vi "DSB Modulation PLL for Graph.vi"() -> ()   [LabVIEW 2013]
uses:
  <vilib>/sound2/lvsound2.llb/Sound File Info (path).vi
  <vilib>/sound2/lvsound2.llb/Sound File Read Open.vi
  <vilib>/sound2/lvsound2.llb/Sound File Read (DBL).vi
  <vilib>/Waveform/WDTOps.llb/WDT Get Waveform Subset DBL.vi
  <vilib>/addons/Modulation/Analog/MT Passband PLL.vi
  <vilib>/express/express analysis/Spectral/Block/exnSpectralBlock spectral measurements RMS poly.vi
  <vilib>/express/express analysis/Spectral/Block/exnSpectralBlock spectral measurements RMS DDT.vi
  <vilib>/express/express analysis/Spectral/XNode/ExpressSpectralMeasurementsBlockNode.xnode
  <vilib>/addons/Modulation/niAMT.lvlib
panel:
  in  "Modulated Signal Source":enum32{"Single Tone", "From File"}(tab)
  in  "ST Frequency":dbl=2000.0 caption="Frequency"
  in  "ST Amplitude":dbl=1.0 caption="Amplitude"
  in  "Resample Rate":dbl=1000000.0 format="%#_6f"
  in  "Duration":dbl=44100.0
  in  "WAV Path":path caption="Path"
  out "DSB Squared":dynamicdata(graph)
  out "Estimated Freq.":dbl caption="Amplitude" format="%#_9g"
  in  "WAV Sample Rate":dbl=44100.0 caption="dt"
  in  "LPF Cut-Off":dbl=50000.0 caption="Lower Cut-Off"
  in  "SNR (dB)":dbl(slide)=30.0 caption="Standard deviation" scale=-20.0..30.0
  out "Comparision":dynamicdata(graph)
  out "Baseband":dynamicdata(graph)
  out "DSB FFT":dynamicdata(graph)
  out "DSB Wave":dynamicdata(graph)
  in  "Carrier Amp.":dbl=1.0 caption="Amplitude"
  in  "stop":bool
  in  "Frequency Offset":dbl(slide) scale=-1000.0..1000.0
  in  "Carrier Freq.":dbl=100000.0 caption="Frequency"
  # "DSB Modulation"
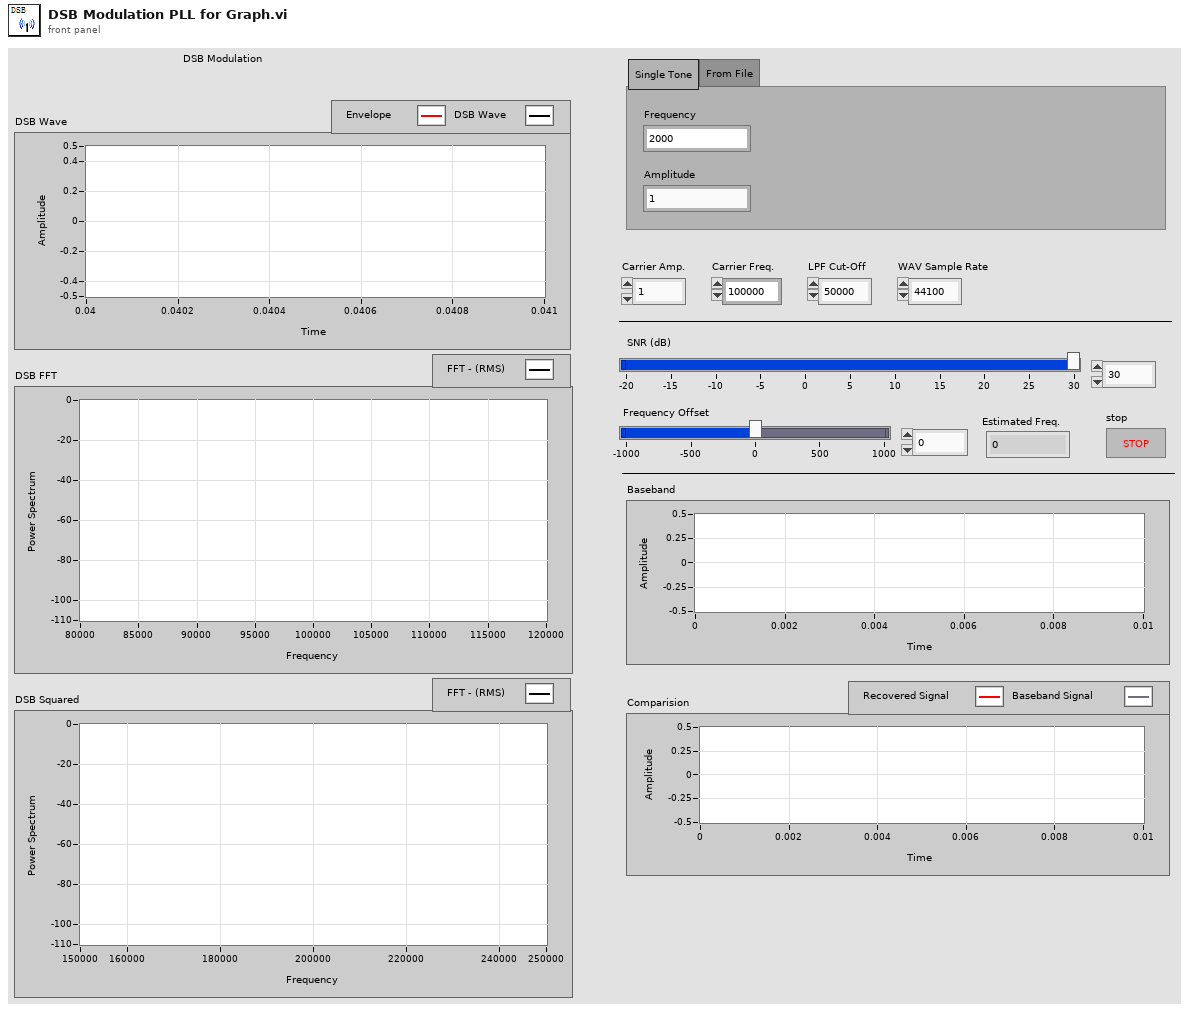
[diagram p1: front panel]
types:
  T1 = typedef "Sound File Refnum.ctl" = refnum<file>
  T2 = cluster{"averaging mode":u16, "weighting mode":u16, "number of averages":u32}
  T3 = cluster{"dB On (F)":bool, "unwrap phase (F)":bool, "convert to degree (F)":bool}
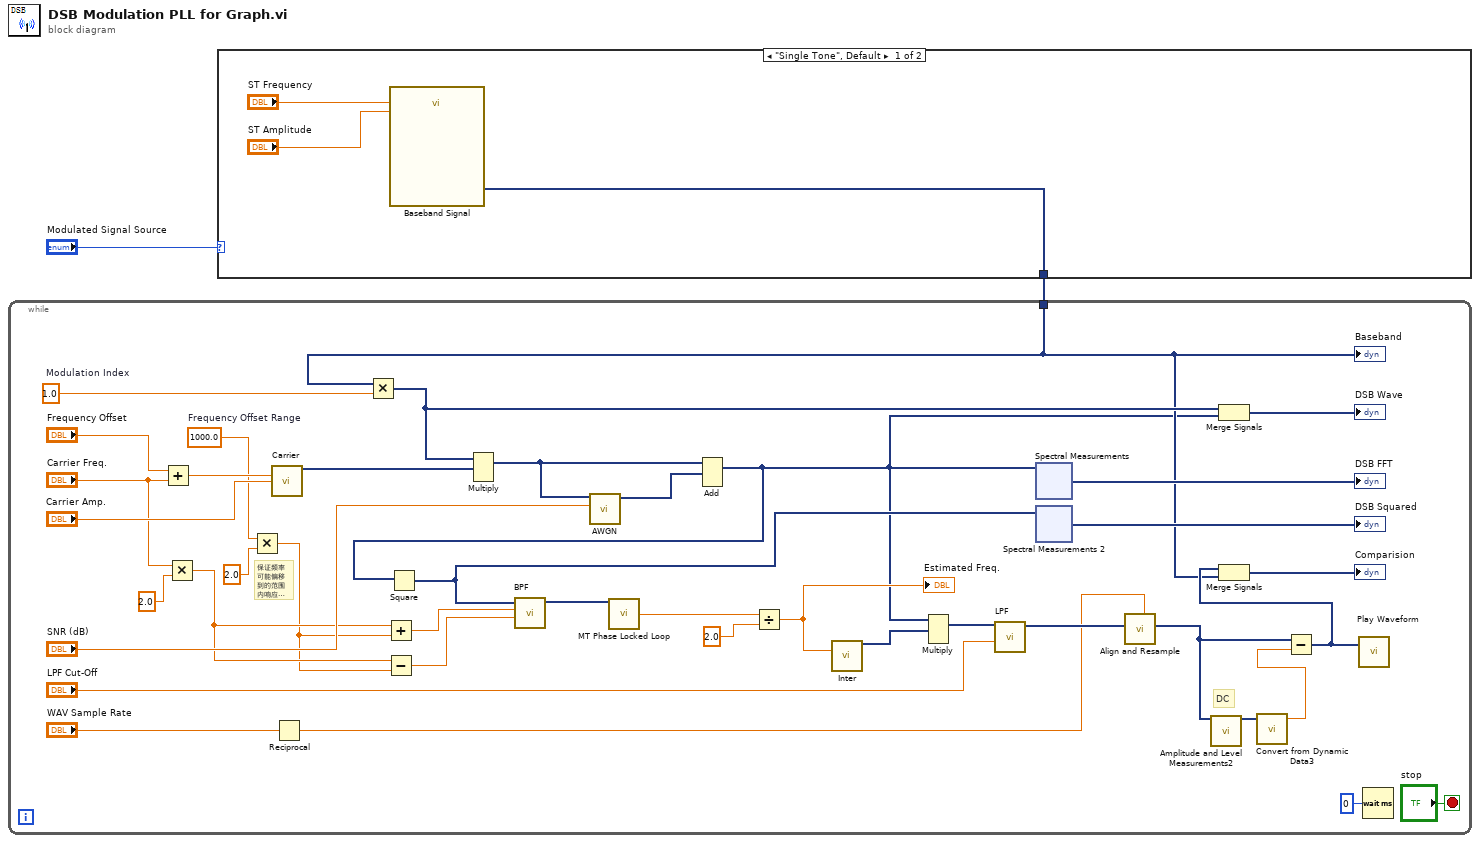
[diagram p0: block diagram]
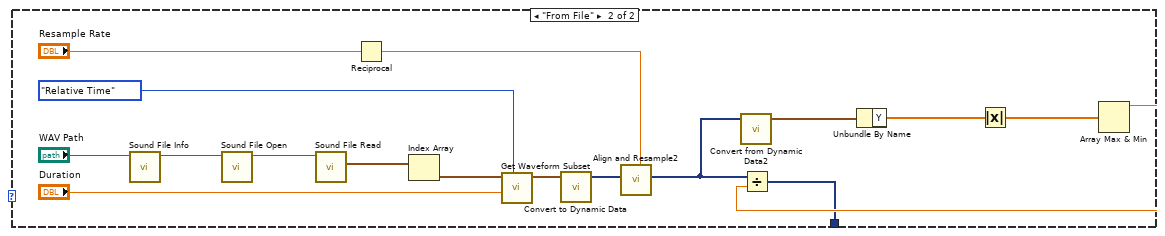
[diagram p2: hidden frame]
diagram:
  n1 = case shown="\"Single Tone\", Default" "Modulated Signal Source" {
    tunnel: [w3 w7] -> w1
    frame "Single Tone", Default {
      n2 = call "Baseband Signal"("Frequency"="ST Frequency", "Amplitude"="ST Amplitude") -> ("Sine"=w3:dynamicdata)  [unwired: 12 in, 1 out]
    }
    frame "From File" {
      n3 = call-poly <vilib>:"Sound File Info.vi"("path"="WAV Path") -> ("path out"=w20:path)  [unwired: 7 in, 3 out]
      n4 = call-poly <vilib>:"Sound File Open.vi"("path"=w20) -> ("sound file refnum"=w22:T1)  [unwired: 9 in, 1 out]
      n5 = call-poly <vilib>:"Sound File Read.vi"("sound file refnum"=w22) -> ("data"=w17:waveform(dbl)[])  [unwired: 6 in, 4 out]
      n6 = Reciprocal(x="Resample Rate") -> (1/x=w13:dbl)
      n7 = Index Array(array=w17) -> (element=w18:waveform(dbl))  [unwired: 1 in]
      n8 = call-poly <vilib>:"Get Waveform Subset.vi"("start/duration format"=enum16{"Relative Time"}."Relative Time", "duration"="Duration", "waveform in"=w18) -> ("waveform out"=w12:waveform(dbl))  [unwired: 3 in, 3 out]
      n9 = call "Convert to Dynamic Data"("Waveform"=w12) -> ("Dynamic Data Type"=w6:dynamicdata)  [unwired: 3 in]
      n10 = call "Align and Resample2"("dt"=w13, "Signals"=w6) -> ("Resampled Signals"=w8:dynamicdata)  [unwired: 7 in, 2 out]
      n11 = call "Convert from Dynamic Data2"("Dynamic Data Type"=w8) -> ("Waveform"=w15:waveform(dbl))  [unwired: 3 in]
      n12 = Unbundle By Name(w15) -> ("Y"=w9:dbl[])
      n13 = Absolute Value(x=w9) -> (abs(x)=w11:dbl[])
      n14 = Array Max & Min(array=w11) -> (max value=w10:dbl)  [unwired: 3 out]
      n15 = Divide(x=w8, y=w10) -> (x/y=w7:dynamicdata)
    }
  }
  n16 = while {
    tunnel: w1 -> [w31]
    stop <- "stop" stop-if-true
    w27 = 1000.0  # Frequency Offset Range
    w56 = 1.0  # Modulation Index
    # "保证频率可能偏移到的范围内响应是平的"
    # "DC"
    n17 = Add(x="Frequency Offset", y="Carrier Freq.") -> (x+y=w55:dbl)
    n18 = Multiply(x="Carrier Freq.", y=2.0) -> (x*y=w35:dbl)
    n19 = Multiply(x=w27, y=2.0) -> (x*y=w28:dbl)
    n20 = call "Carrier"("Frequency"=w55, "Amplitude"="Carrier Amp.") -> ("Sine"=w52:dynamicdata)  [unwired: 12 in, 1 out]
    n21 = Reciprocal(x="WAV Sample Rate") -> (1/x=w45:dbl)
    n22 = Multiply(x=w31, y=w56) -> (x*y=w51:dynamicdata)
    n23 = Add(x=w35, y=w28) -> (x+y=w33:dbl)
    n24 = Subtract(x=w35, y=w28) -> (x-y=w32:dbl)
    n25 = Multiply(1:w52, 2:w51) -> (0:w50:dynamicdata)  [unwired: 1 in, 1 out]
    n26 = call "AWGN.vi"("SNR (dB)"="SNR (dB)", "Dynamic Data"=w50) -> ("DC with Gaussian Noise"=w49:dynamicdata)  [unwired: 9 in]
    n27 = Add(1:w49, 2:w50) -> (0:w23:dynamicdata)  [unwired: 1 in, 1 out]
    n28 = Square(x=w23) -> (x^2=w30:dynamicdata)
    n29 = call "BPF"("Lower Cut-Off"=w32, "Upper Cut-Off"=w33, "Signal"=w30) -> ("Filtered Signal"=w24:dynamicdata)  [unwired: 7 in, 1 out]
    n30 = call-poly <vilib>:"MT Phase Locked Loop.vi"("passband waveform"=w24) -> ("estimated carrier frequency (Hz)"=w25:dbl)  [unwired: 10 in, 4 out]
    n31 = Divide(x=w25, y=2.0) -> (x/y=w26:dbl)
    "Estimated Freq." <- w26
    n32 = call "Inter"("Frequency"=w26) -> ("Sine"=w39:dynamicdata)  [unwired: 13 in, 1 out]
    n33 = Multiply(1:w39, 2:w23) -> (0:w40:dynamicdata)  [unwired: 1 in, 1 out]
    n34 = call "LPF"("Lower Cut-Off"="LPF Cut-Off", "Signal"=w40) -> ("Filtered Signal"=w47:dynamicdata)  [unwired: 8 in, 1 out]
    n35 = xnode ("Spectral Measurements")("Signals"=w23) -> ("FFT - (RMS)"=→"DSB FFT":dynamicdata)  [unwired: 1 in, 2 out]
    n36 = xnode ("Spectral Measurements 2")("Signals"=w30) -> ("FFT - (RMS)"=→"DSB Squared":dynamicdata)  [unwired: 1 in, 2 out]
    n37 = call "Align and Resample"("dt"=w45, "Signals"=w47) -> ("Resampled Signals"=w59:dynamicdata)  [unwired: 7 in, 2 out]
    n38 = call "Amplitude and Level Measurements2"("Signals"=w59) -> ("Mean (DC)"=w61:dynamicdata)  [unwired: 13 in, 1 out]
    n39 = Merge Signals(w51, w23) -> (→"DSB Wave":dynamicdata)
    n40 = call "Convert from Dynamic Data3"("Dynamic Data Type"=w61) -> ("Scalar"=w58:dbl)  [unwired: 3 in]
    n41 = Subtract(x=w59, y=w58) -> (x-y=w43:dynamicdata)
    n42 = Merge Signals(w43, w31) -> (→"Comparision":dynamicdata)
    n43 = call "Play Waveform"("Data"=w43) -> ()  [unwired: 18 in, 1 out]
    n44 = Wait (ms)(milliseconds to wait=u32 0) -> ()  [unwired: 1 out]
    "Baseband" <- w31
  }
